vi "libssh2_userauth_password.vi"(8 "error in (no error)":errorcluster, 9 "password":string, 10 "username":string, 11 "session":T1) -> (0 "error out":errorcluster)   [LabVIEW 2013, in "libssh2.lvlib"]
doc: "Authenticates a session with username and password."
uses:
  libssh2.lvlib
  Session Refnum.ctl
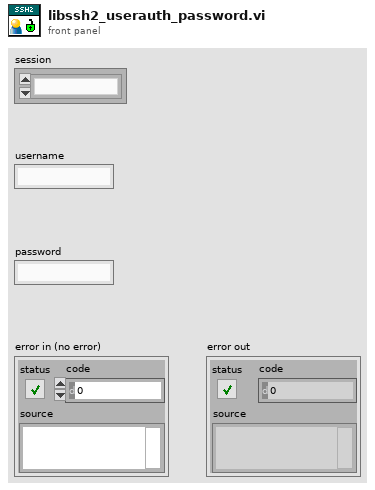
[diagram p1: front panel]
types:
  T1 = typedef "libssh2.lvlib/Session Refnum.ctl" = refnum<k1>
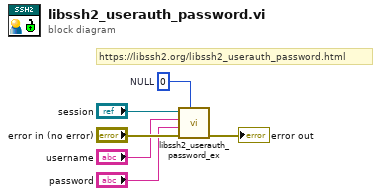
[diagram p0: block diagram]
diagram:
  w1 = u64 0  # NULL
  # "https://libssh2.org/libssh2_userauth_password.html"
  n1 = call "libssh2_userauth_password_ex.vi"("passwd_change_cb"=w1, "error in (no error)"="error in (no error)", "password"="password", "username"="username", "session"="session") -> ("error out"=→"error out":errorcluster)  [unwired: 6 in]
